vi "CreateSensorSession.vi"(8 "error in (no error)":errorcluster, 11 "SiemensDigitalEnergyMeter in":refnum<class "SiemensDigitalEnergyMeter.lvclass">) -> (0 "error out":errorcluster, 3 "SiemensDigitalEnergyMeter out":refnum<class "SiemensDigitalEnergyMeter.lvclass">)   [LabVIEW 2018, in "SensorPlugins.lvlib" / "SiemensDigitalEnergyMeter.lvclass"]
doc: "This VI opens a communication link between the application and the Siemens Digital Energy Meter using an IP address and a port number."
uses:
  SiemensDigitalEnergyMeter.lvclass
  <vilib>/Modbus/master/Create Master Instance (TCP).vi
  <vilib>/Modbus/master/Modbus Master.lvclass
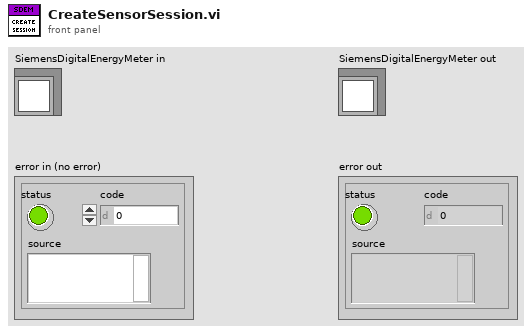
[diagram p1: front panel]
types:
  T1 = typedef "SensorPlugins.lvlib/SiemensDigitalEnergyMeter.lvclass/SiemensDigitalEnergyMeterControls.ctl" = cluster{"Measurement(s)":u16[], "IP Address":string, "Port (502)":u16, "Configuration Commands":string, "Use Measurement Commands Text Box?":bool, "Measurement Commands":string, "Connected?":bool}[]
  T2 = cluster{"Measurement(s)":u16[], "IP Address":string, "Port (502)":u16, "Configuration Commands":string, "Use Measurement Commands Text Box?":bool, "Measurement Commands":string, "Connected?":bool}
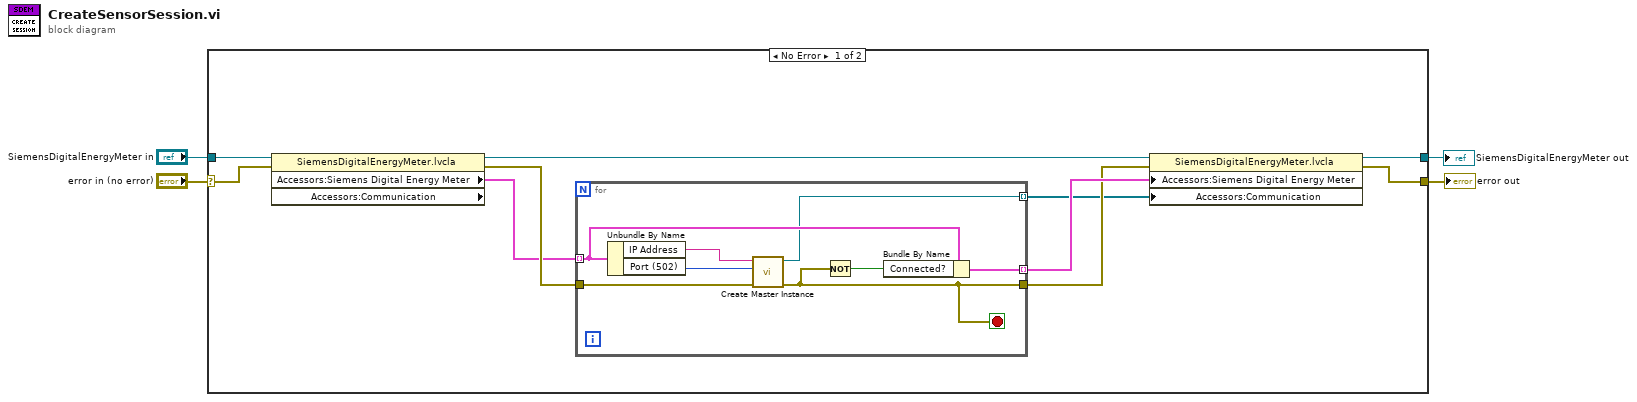
[diagram p0: block diagram]
diagram:
  n1 = case shown="No Error" "error in (no error)" {
    selector: "error in (no error)" -> [w13 w23]
    tunnel: "SiemensDigitalEnergyMeter in" -> [w14 w24]
    tunnel: [w10 w24] -> w2
    tunnel: [w6 w23] -> w1
    frame No Error {
      n2 = property class="SiemensDigitalEnergyMeter.lvcla" props=["Accessors:Siemens Digital Energy Meter", "Accessors:Communication"](reference=w14, error in=w13) -> (reference out=w9:refnum<class "SiemensDigitalEnergyMeter.lvclass">, error out=w12:errorcluster, "Accessors:Siemens Digital Energy Meter"=w11:T1)  [unwired: 1 out]
      n3 = for {
        tunnel: w12 -> [w22]
        tunnel: [w17] -> w7
        tunnel: w11 -> [w19] mode=indexing
        tunnel: [w18] -> w8 mode=indexing
        tunnel: [w15] -> w5 mode=indexing
        stop <- w17 stop-if-true
        n4 = Unbundle By Name(w19) -> ("IP Address"=w21:string, "Port (502)"=w20:u16)
        n5 = call-poly <vilib>:"Create Master Instance.vi"("error in (no error)"=w22, "port (502)"=w20, "address"=w21) -> ("error out"=w17:errorcluster, "TCP master instance"=w15:refnum<class "Modbus Master.lvclass">)  [unwired: 7 in]
        n6 = Not(x=w17) -> (.not. x?=w16:bool)
        n7 = Bundle By Name(cluster=w19, "Connected?"=w16) -> (w18:T2)
      }
      n8 = property class="SiemensDigitalEnergyMeter.lvcla"(reference=w9, error in=w7, "Accessors:Siemens Digital Energy Meter"=w8, "Accessors:Communication"=w5) -> (reference out=w10:refnum<class "SiemensDigitalEnergyMeter.lvclass">, error out=w6:errorcluster)
    }
    frame Error {
    }
  }
  "error out" <- w1
  "SiemensDigitalEnergyMeter out" <- w2
